vi "Compare Datatype.vi"(8 "错误输入（无错误）":errorcluster, 10 "Type 2":variant, 11 "Type 1":variant) -> (0 "错误输出":errorcluster, 3 "Compare Result":enum16{"Same", "Convert", "Not Same"}(ring))   [LabVIEW 2012, in "Application.lvlib"]
uses:
  Application.lvlib
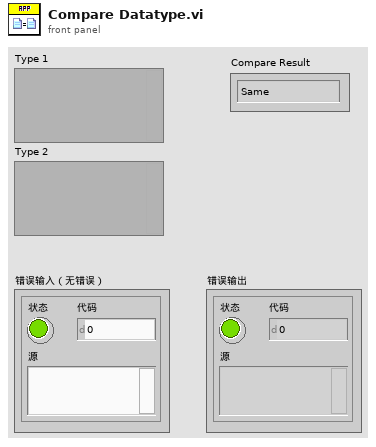
[diagram p1: front panel]
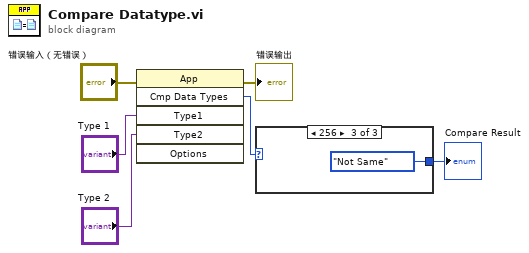
[diagram p0: block diagram]
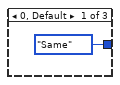
[diagram p2: hidden frame]
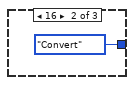
[diagram p3: hidden frame]
diagram:
  n1 = invoke class="App" method="Cmp Data Types"(error in="错误输入（无错误）", "Type1"="Type 1", "Type2"="Type 2") -> (error out=→"错误输出":errorcluster, "Compare Data Types"=w2:i32)  [unwired: 3 in, 4 out]
  n2 = case shown="256" w2 {
    tunnel: [enum16{"Same", "Convert", "Not Same"}."Same" ("枚举") enum16{"Same", "Convert", "Not Same"}."Convert" ("枚举") enum16{"Same", "Convert", "Not Same"}."Not Same" ("枚举")] -> w1
    frame 0, Default {
    }
    frame 16 {
    }
    frame 256 {
    }
  }
  "Compare Result" <- w1
